vi "Continue Z Scan.vi"(7 "Error Signal Notifier":refnum<notifier>, 8 "error in (no error)":errorcluster, 9 "Automation State In":T1, 10 "Automation Queue":refnum<queue>, 11 "UI Queue":refnum<queue>) -> (0 "error out":errorcluster, 1 "Automation State Out":T1, 2 "Keep looping?":bool)   [LabVIEW 2013, in "Automation.lvlib"]
uses:
  Automation.lvlib
  Automation State.ctl
  Zscan Settings.ctl
  support/Message Queue/Message Cluster.ctl
  Feedback/Error Signal.ctl
  support/Message Queue/Enqueue Message (Single).vi
  support/Message Queue/Message Queue.lvlib
  Feedback/Feedback.lvlib
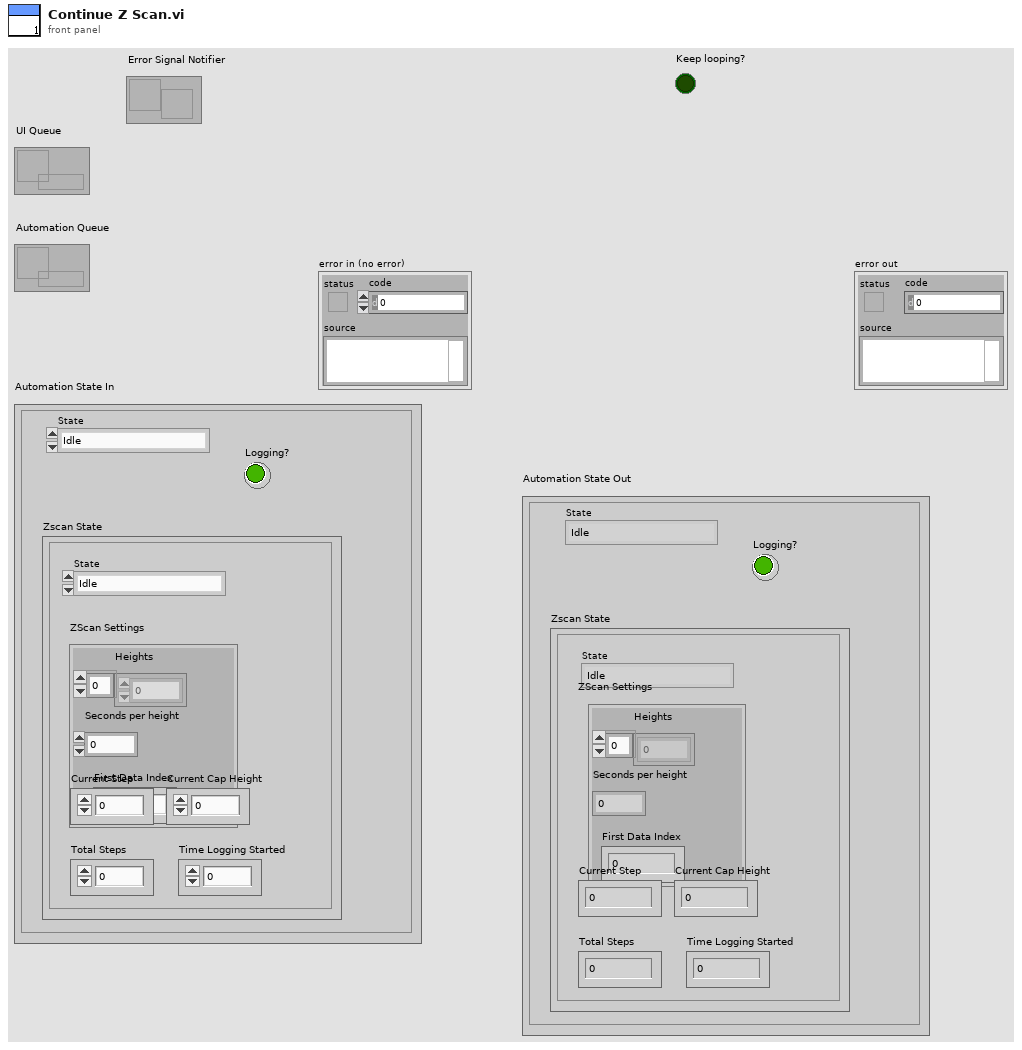
[diagram p1: front panel]
types:
  T1 = typedef "Automation.lvlib/Automation State.ctl" = cluster{"State":enum16{"Idle", "Zscan"}, "Logging?":bool, "Zscan State":cluster{"State":enum16{"Idle", "Waiting for lock", "Waiting for acquisition"}, "ZScan Settings":T2, "Current Step":i32, "Current Cap Height":dbl, "Total Steps":i32, "Time Logging Started":dbl}}
  T2 = typedef "Automation.lvlib/Zscan Settings.ctl" = cluster{"Heights":dbl[], "Seconds per height":i32, "First Data Index":i32}
  T3 = cluster{"State":enum16{"Idle", "Waiting for lock", "Waiting for acquisition"}, "ZScan Settings":T2, "Current Step":i32, "Current Cap Height":dbl, "Total Steps":i32, "Time Logging Started":dbl}
  T4 = enum16{"Idle", "Waiting for lock", "Waiting for acquisition"}
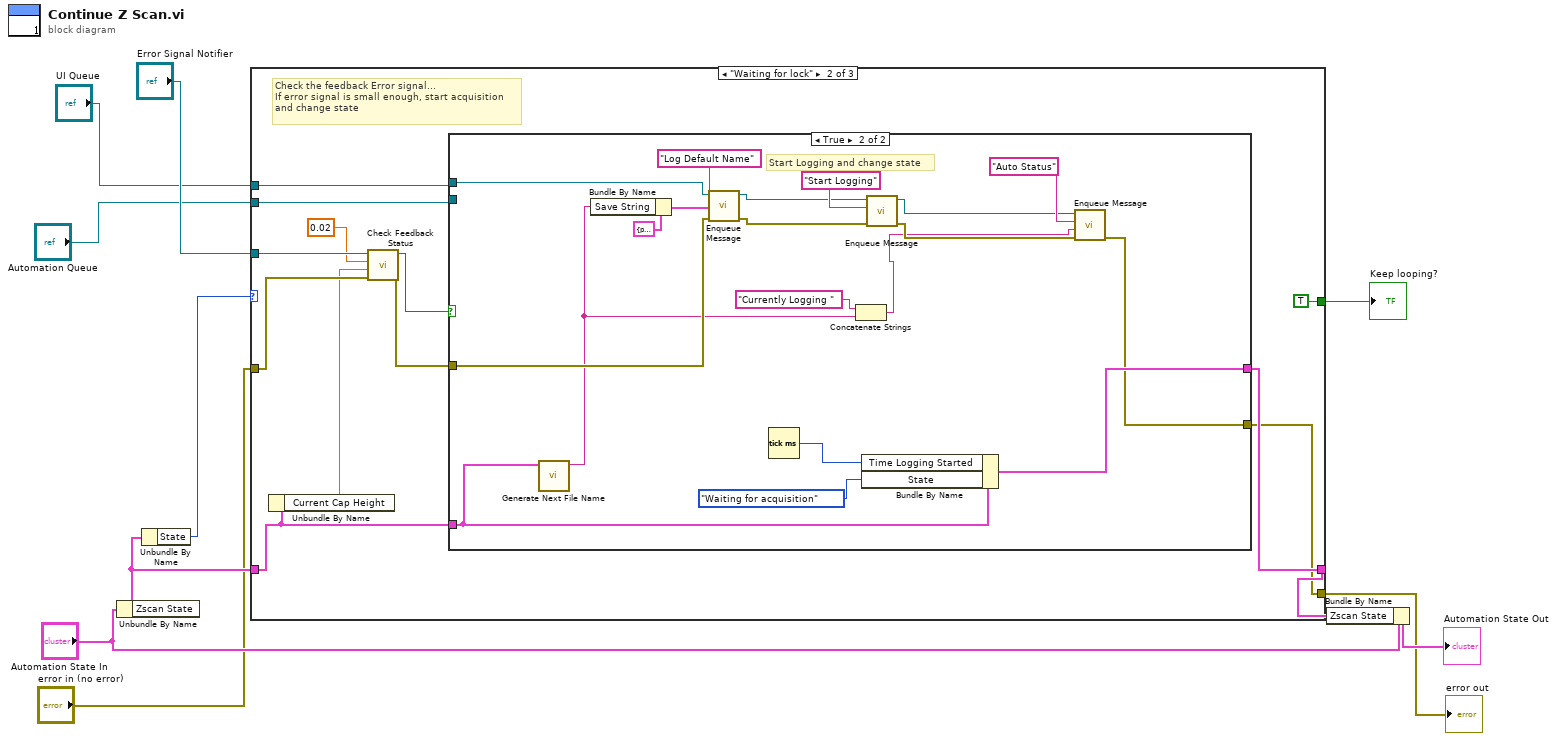
[diagram p0: block diagram]
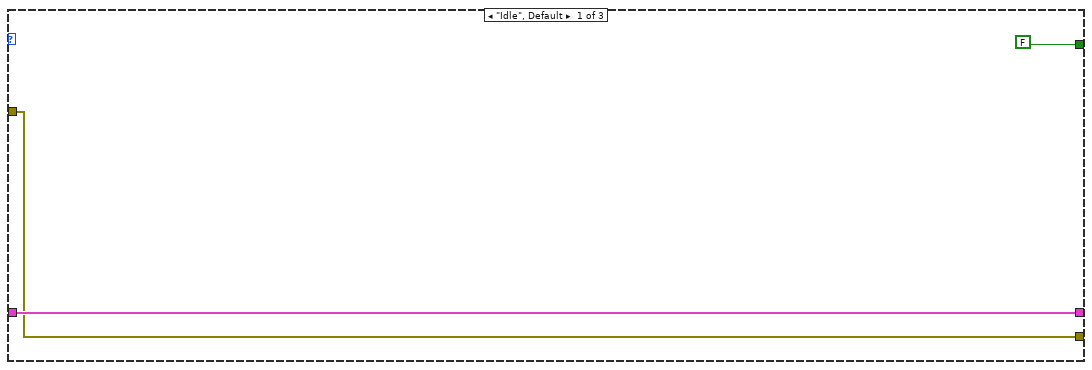
[diagram p2: hidden frame]
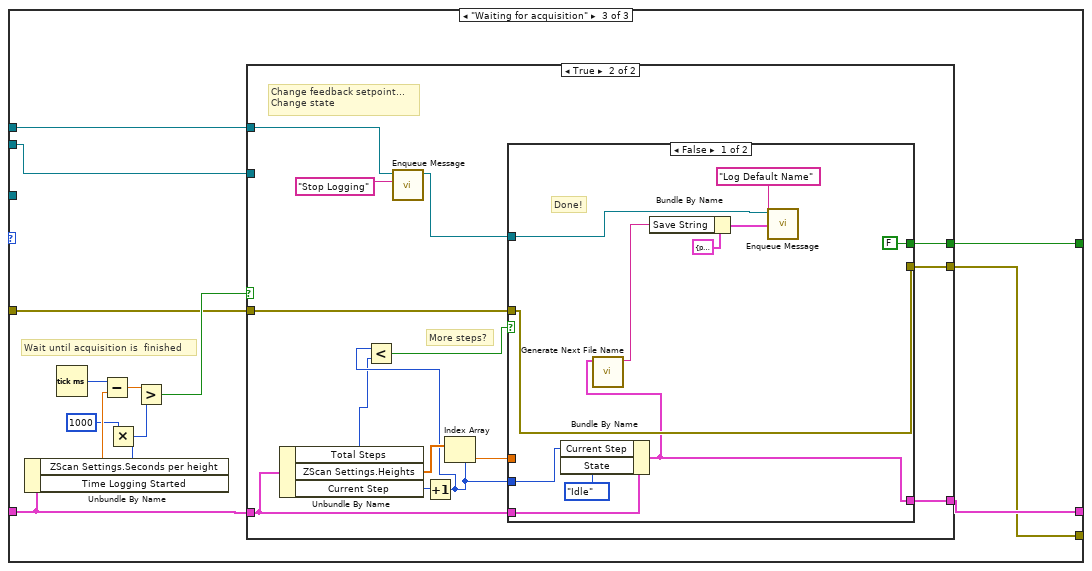
[diagram p4: hidden frame]
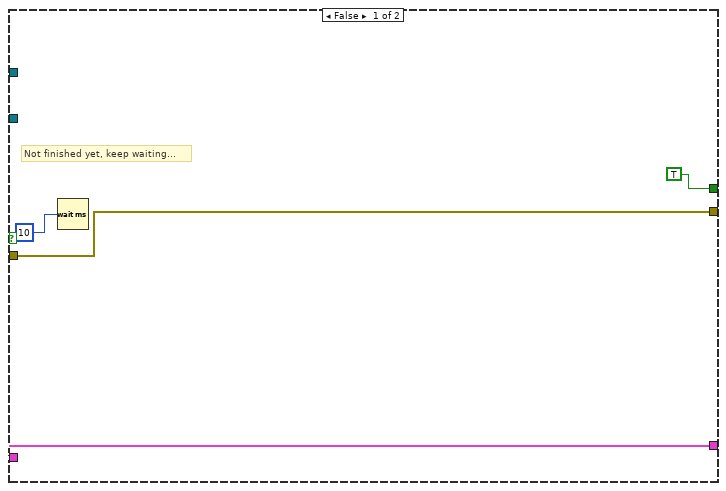
[diagram p5: hidden frame]
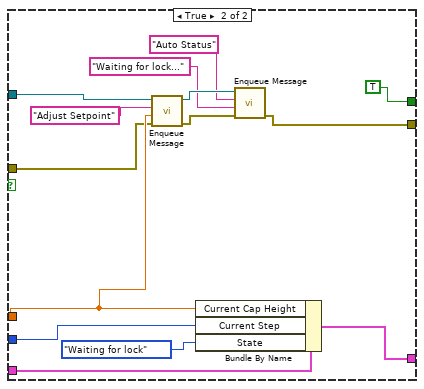
[diagram p6: hidden frame]
diagram:
  n1 = Unbundle By Name("Automation State In") -> ("Zscan State"=w8:T3)
  n2 = Unbundle By Name(w8) -> ("State"=w7:T4)
  n3 = case shown="\"Waiting for lock\"" w7 {
    tunnel: [w14 w23 w53] -> w9
    tunnel: w8 -> [w14 w16 w54]
    tunnel: "Error Signal Notifier" -> [_ w26 _]
    tunnel: "Automation Queue" -> [_ w22 w49]
    tunnel: "error in (no error)" -> [w13 w18 w51]
    tunnel: [w13 w21 w50] -> w3
    tunnel: "UI Queue" -> [_ w19 w52]
    tunnel: [FALSE ("Keep looping?") TRUE ("Keep looping?") w48] -> w1
    frame "Idle", Default {
    }
    frame "Waiting for lock" {
      # "Check the feedback Error signal...\nIf error signal is small enough, start acquisition\nand change state"
      n4 = Unbundle By Name(w16) -> ("Current Cap Height"=w15:dbl)
      n5 = call "Check Feedback Status.vi"("error in (no error)"=w18, "Current Set Height"=w15, "Threshold (um)"=0.02, "Error Signal Notifier"=w26) -> ("error out"=w17:errorcluster, "Locked"=w24:bool)  [unwired: 6 in]
      n6 = case shown="True" w24 {
        tunnel: w16 -> [w28 w33]
        tunnel: [w28 w47] -> w23
        tunnel: w22 -> [_ _]
        tunnel: w17 -> [w27 w36]
        tunnel: [w27 w41] -> w21
        tunnel: w19 -> [_ w29]
        frame False {
          # "If not locked, keep looping"
        }
        frame True {
          # "Start Logging and change state"
          n7 = call "Generate Next File Name.vi"("Zscan State"=w33) -> ("String"=w31:string)  [unwired: 10 in]
          n8 = Bundle By Name(cluster=cluster{"Save Path":path, "Save String":string} {"Save Path"=path "", "Save String"=""} ("output cluster"), "Save String"=w31) -> (w34:cluster{"Save Path":path, "Save String":string})
          n9 = call-poly "Enqueue Message.vi"("error in (no error)"=w36, "Message Data"=w34, "Message"="Log Default Name", "Message Queue"=w29) -> ("error out"=w38:errorcluster, "dup Message Queue"=w37:refnum<queue>)  [unwired: 6 in]
          n10 = Tick Count (ms)() -> (millisecond timer value=w44:u32)
          n11 = Concatenate Strings("Currently Logging " ("Message"), w31) -> (w30:string)
          n12 = Bundle By Name(cluster=w33, "Time Logging Started"=w44, "State"=T4."Waiting for acquisition") -> (w47:T3)
          n13 = call-poly "Enqueue Message.vi"("error in (no error)"=w38, "Message"="Start Logging", "Message Queue"=w37) -> ("error out"=w42:errorcluster, "dup Message Queue"=w40:refnum<queue>)  [unwired: 7 in]
          n14 = call-poly "Enqueue Message.vi"("error in (no error)"=w42, "Message Data"=w30, "Message"="Auto Status", "Message Queue"=w40) -> ("error out"=w41:errorcluster)  [unwired: 6 in, 1 out]
        }
      }
    }
    frame "Waiting for acquisition" {
      # "Wait until acquisition is  finished"
      n15 = Unbundle By Name(w54) -> ("ZScan Settings.Seconds per height"=w58:i32, "Time Logging Started"=w60:dbl)
      n16 = Tick Count (ms)() -> (millisecond timer value=w61:u32)
      n17 = Subtract(x=w61, y=w60) -> (x-y=w59:dbl)
      n18 = Multiply(x=1000, y=w58) -> (x*y=w56:i32)
      n19 = Greater?(x=w59, y=w56) -> (0:w55:bool)
      n20 = case shown="True" w55 {
        tunnel: w54 -> [w64 w78]
        tunnel: [w64 w79] -> w53
        tunnel: w52 -> [_ w67]
        tunnel: w51 -> [w63 w74]
        tunnel: [w63 w73] -> w50
        tunnel: w49 -> [_ _]
        tunnel: [TRUE ("Keep looping?") w68] -> w48
        frame False {
          # "Not finished yet, keep waiting..."
          n21 = Wait (ms)(milliseconds to wait=u32 10) -> ()  [unwired: 1 out]
        }
        frame True {
          # "More steps?"
          # "Change feedback setpoint...\nChange state"
          n22 = Unbundle By Name(w78) -> ("Total Steps"=w71:i32, "ZScan Settings.Heights"=w76:dbl[], "Current Step"=w77:i32)
          n23 = call-poly "Enqueue Message.vi"("Message"="Stop Logging", "Message Queue"=w67) -> ("dup Message Queue"=w66:refnum<queue>)  [unwired: 8 in, 1 out]
          n24 = Increment(x=w77) -> (x+1=w72:i32)
          n25 = Less?(x=w72, y=w71) -> (x < y?=w70:bool)
          n26 = Index Array(array=w76, index=w72) -> (element=w75:dbl)
          n27 = case shown="False" w70 {
            tunnel: [w80 w103] -> w79
            tunnel: w78 -> [w88 w102]
            tunnel: w72 -> [w81 w101]
            tunnel: w66 -> [w83 w99]
            tunnel: w75 -> [_ w98]
            tunnel: w74 -> [w90 w97]
            tunnel: [w90 w93] -> w73
            tunnel: [FALSE ("Keep looping?") TRUE ("Keep looping?")] -> w68
            frame False {
              # "Done!"
              n28 = Bundle By Name(cluster=w88, "Current Step"=w81, "State"=T4."Idle") -> (w80:T3)
              n29 = call "Generate Next File Name.vi"("Zscan State"=w80) -> ("String"=w82:string)  [unwired: 10 in]
              n30 = Bundle By Name(cluster=cluster{"Save Path":path, "Save String":string} {"Save Path"=path "", "Save String"=""} ("output cluster"), "Save String"=w82) -> (w84:cluster{"Save Path":path, "Save String":string})
              n31 = call-poly "Enqueue Message.vi"("Message Data"=w84, "Message"="Log Default Name", "Message Queue"=w83) -> ()  [unwired: 7 in, 2 out]
            }
            frame True {
              n32 = call-poly "Enqueue Message.vi"("error in (no error)"=w97, "Message Data"=w98, "Message"="Adjust Setpoint", "Message Queue"=w99) -> ("error out"=w94:errorcluster, "dup Message Queue"=w95:refnum<queue>)  [unwired: 6 in]
              n33 = Bundle By Name(cluster=w102, "Current Cap Height"=w98, "Current Step"=w101, "State"=T4."Waiting for lock") -> (w103:T3)
              n34 = call-poly "Enqueue Message.vi"("error in (no error)"=w94, "Message Data"="Waiting for lock..." ("Message"), "Message"="Auto Status", "Message Queue"=w95) -> ("error out"=w93:errorcluster)  [unwired: 6 in, 1 out]
            }
          }
        }
      }
    }
  }
  "error out" <- w3
  "Keep looping?" <- w1
  n35 = Bundle By Name(cluster="Automation State In", "Zscan State"=w9) -> (→"Automation State Out":T1)
